vi "CreateModbusURLs.vi"(8 "error in (no error)":errorcluster, 9 "Start Address":u16, 10 "Base Addres URL":string, 11 "Timing Groups":refnum<class "TimingGrp.lvclass">) -> (0 "error out":errorcluster, 3 "Timing Groups":refnum<class "TimingGrp.lvclass">)   [LabVIEW 2012, in "Configuration Grandmaster.lvlib" / "TimingGrp.lvclass"]
uses:
  TimingGrp.lvclass
  Custom Ctrls/Modbus Address Header.ctl
  TimingGrp.lvclass/TimingGrp.ctl
  Class Chan Group/ChanGrp.lvclass
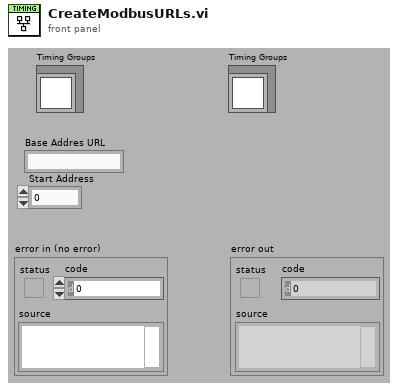
[diagram p1: front panel]
types:
  T1 = typedef "Modbus Address Header.ctl" = string
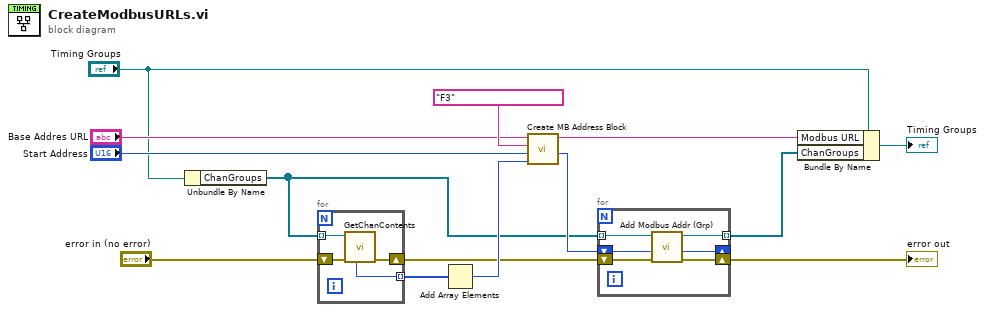
[diagram p0: block diagram]
diagram:
  n1 = Unbundle By Name("Timing Groups") -> ("ChanGroups"=w1:refnum<class "ChanGrp.lvclass">[])
  n2 = for {
    tunnel: [w17] -> w12 mode=indexing
    tunnel: w1 -> [w18] mode=indexing
    shift-right: [w15] -> w3
    shift-left: "error in (no error)" -> [w16]
    n3 = call "GetChanContents.vi"("error in"=w16, "ChanGrp.lvclass"=w18) -> ("error out"=w15:errorcluster, "Num Modbus Enbld"=w17:i16)  [unwired: 3 in, 5 out]
  }
  n4 = Add Array Elements(numeric array=w12) -> (sum=w13:i16)
  n5 = call "Create MB Address Block.vi"("Number of Registers in Block"=w13, "Start Address"="Start Address", "Modbus Address Type"=T1 "F3", "Base Address URL"="Base Addres URL") -> ("Starting Address (SGL)"=w11:i32, "Modbus URL"=w7:string)  [unwired: 6 in]
  n6 = for {
    shift-right: [w22] -> _
    shift-left: w11 -> [w23]
    tunnel: w1 -> [w24] mode=indexing
    tunnel: [w21] -> w6 mode=indexing
    shift-right: [w19] -> w2
    shift-left: w3 -> [w20]
    n7 = call "Add Modbus Addr (Grp).vi"("error in"=w20, "Starting Address (SGL)"=w23, "ChanGrp.lvclass"=w24) -> ("error our"=w19:errorcluster, "Next Address (SGL)"=w22:i32, "ChanGrp.lvclass"=w21:refnum<class "ChanGrp.lvclass">)  [unwired: 6 in]
  }
  "error out" <- w2
  n8 = Bundle By Name(cluster="Timing Groups", "Modbus URL"=w7, "ChanGroups"=w6) -> (→"Timing Groups":refnum<class "TimingGrp.lvclass">)
